vi "getHPSubnet.vi"(8 "error in (no error)":errorcluster, 11 "ILCCommunications in":refnum<class "ILCCommunications.lvclass">) -> (0 "error out":errorcluster, 2 "Modbus":refnum<class "IModbus.lvclass">, 3 "ILCCommunications out":refnum<class "ILCCommunications.lvclass">)   [LabVIEW 2016, in "ILCCommunications.lvclass"]
uses:
  ILCCommunications.lvclass
  Common_RT_Modbus/IModbus/IModbus.lvclass
  ILCCommunications.lvclass/ILCCommunications.ctl
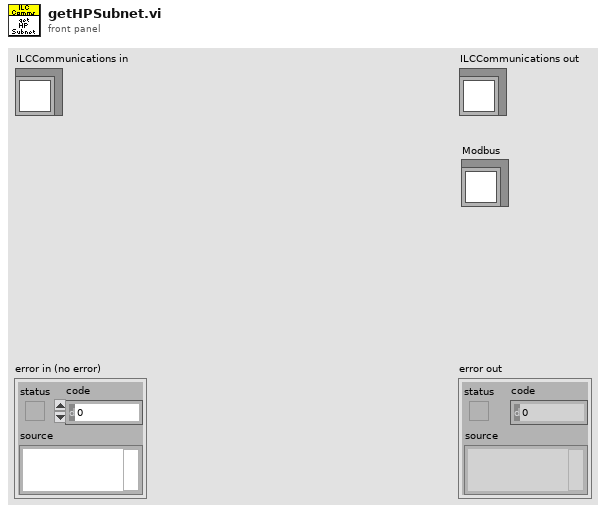
[diagram p1: front panel]
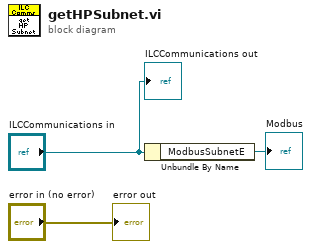
[diagram p0: block diagram]
diagram:
  n1 = Unbundle By Name("ILCCommunications in") -> ("ModbusSubnetE"=→"Modbus":refnum<class "IModbus.lvclass">)
  "error out" <- "error in (no error)"
  "ILCCommunications out" <- "ILCCommunications in"
